vi "Test.vi"(11 "file path (dialog if empty)":path) -> (3 "Last row":dbl[](array[numeric]))   [LabVIEW 2019]
uses:
  <vilib>/Utility/file.llb/Read Delimited Spreadsheet (DBL).vi
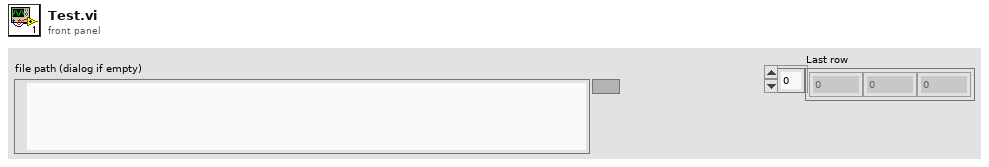
[diagram p1: front panel]
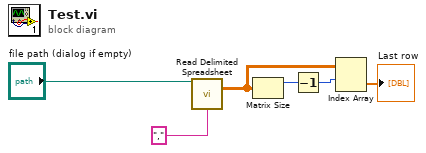
[diagram p0: block diagram]
diagram:
  n1 = call-poly <vilib>:"Read Delimited Spreadsheet.vi"("file path (dialog if empty)"="file path (dialog if empty)", "delimiter (\\t)"="," ("delimiter (\\t)")) -> ("all rows"=w4:dbl[][])  [unwired: 8 in, 5 out]
  n2 = Matrix Size(0:w4) -> (1:w1:i32)  [unwired: 1 out]
  n3 = Decrement(x=w1) -> (x-1=w2:i32)
  n4 = Index Array(array=w4, index (row)=w2) -> (element=→"Last row":dbl[])  [unwired: 1 in]
